vi "FPGA Server v2.vi"() -> ()   [LabVIEW 2013]
doc: "This is the FPGA server for the sbRIO for the open-path cavity ring down."
uses:
  <vilib>/eio/EIONode/EIONode.xnode
  <vilib>/rvi/eio/common/nirviEmuTemplateMethod_errors.vi
  <vilib>/rvi/DataTransferAndStorage/Container/XNode/niFpgaContainer.xnode
  <vilib>/Platform/TimedLoop/XDataNode/XDataNode.xnode
  <vilib>/Platform/TimedLoop/XDataNode/nitl_modes.ctl
  <vilib>/Platform/TimedLoop/XDataNode/XDNodeRunTimeDep.lvlib
  <vilib>/Platform/TimedLoop/XDataNode/wakeup.ctl
  <vilib>/Platform/TimedLoop/XDataNode/timing_clust.ctl
  <vilib>/rvi/Memory/Memory_Emulation/nirvimemoryFastEmulation.vi
  <vilib>/rvi/Memory/Memory_Emulation/nirvimemoryEmulation.vi
  <vilib>/rvi/FIFO/Fifo_Resource/nirvififoEmulationRead.vi
  <vilib>/rvi/FIFO/Fifo_Resource/nirvififoEmulationWrite.vi
  <vilib>/rvi/interface/RandomDataEmulation/nirviRandomDataFpgaReadWriteTemplate.vi
  <vilib>/rvi/FXPMathLib/FxpMul/XNode/nifxpmath_Multiplier.xnode
  <vilib>/rvi/FXPMathLib/sim/FxpSim.dll
panel:
  out "LaserOFF?":bool
  in  "Cylce (ticks)":u32=40000
  in  "Sample (ticks)":u32=8000
  out "DataRead":bool
  out "dataready":bool
  out "NewData":u16
  out "NumElements":u32
  out "Samps":u64
  in  "Stop":bool
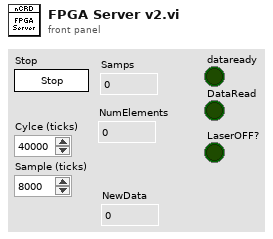
[diagram p1: front panel]
types:
  T1 = typedef "XDNodeRunTimeDep.lvlib/timing_clust.ctl" = cluster{"Expected End [f-1]":u64, "Actual End [f-1]":u64, "Finished Late? [f-1]":bool, "Expected End [i-1]":u64, "Actual End [i-1]":u64, "Finished Late? [i-1]":bool, "Expected Start [i]":u64, "Actual Start [i]":u64, "Expected Start [f]":u64, "Actual Start [f]":u64, "Source Name":string, "Structure Name":string, "Period":i64, "Deadline":i64, "Offset":i64, "Start":i64, "Priority":i32, "Timeout":i32, "Mode":T2, "Wakeup Reason":T3, "Error":errorcluster, "Source Type":string, "Secondary Source Type":string, "Global End Time":u64, "Global Start Time":u64, "Frame Duration":u64, "Iteration Duration":u64, "Assigned CPU":i32, "I/O Scan Engine Mode":u32}
  T2 = typedef "XDNodeRunTimeDep.lvlib/nitl_modes.ctl" = enum32{"No Change", "Process missed periods, maintain original phase", "Discard missed periods, maintain original phase", "Process missed periods, ignore original phase", "Discard missed periods, ignore original phase"}
  T3 = typedef "XDNodeRunTimeDep.lvlib/wakeup.ctl" = enum32{"Normal", "Aborted", "Asynchronous wakeup", "Timing source error", "Timed loop error", "Timeout"}
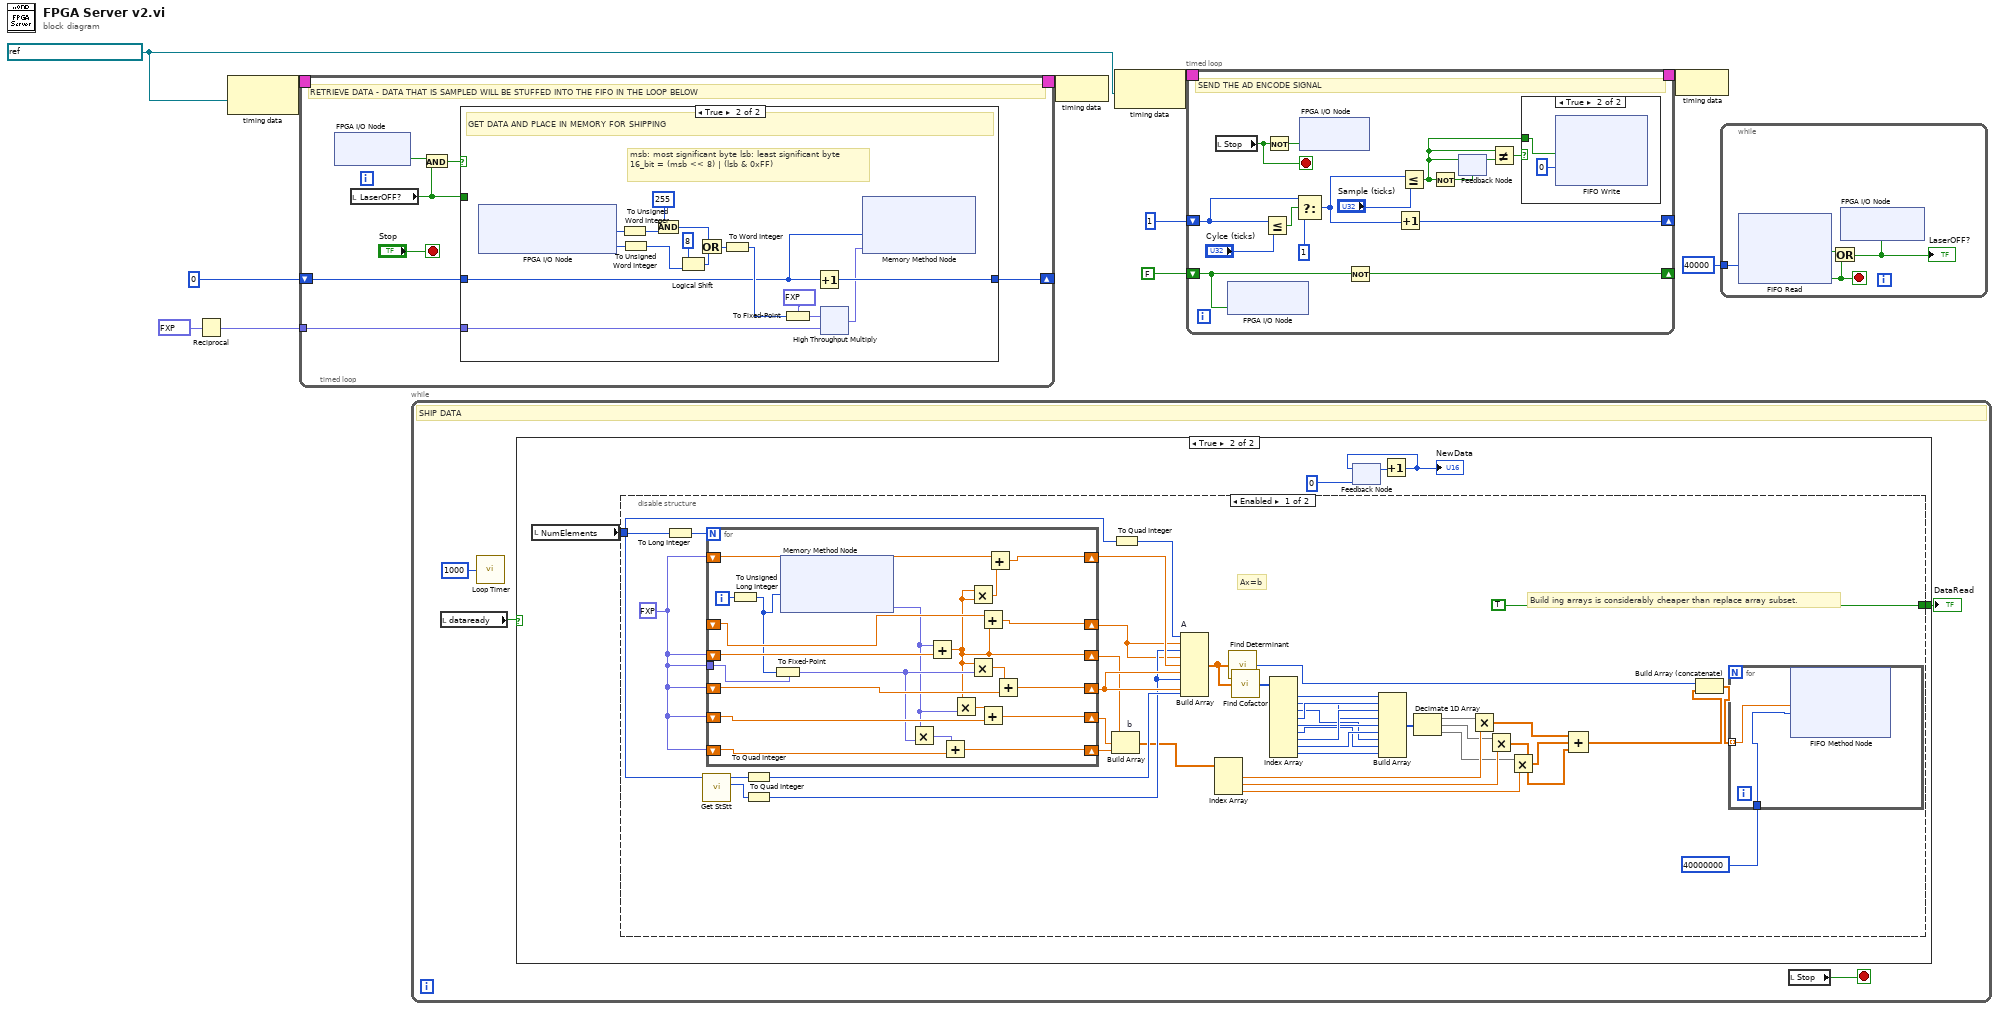
[diagram p0: block diagram]
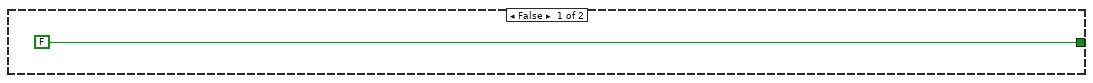
[diagram p2: hidden frame]
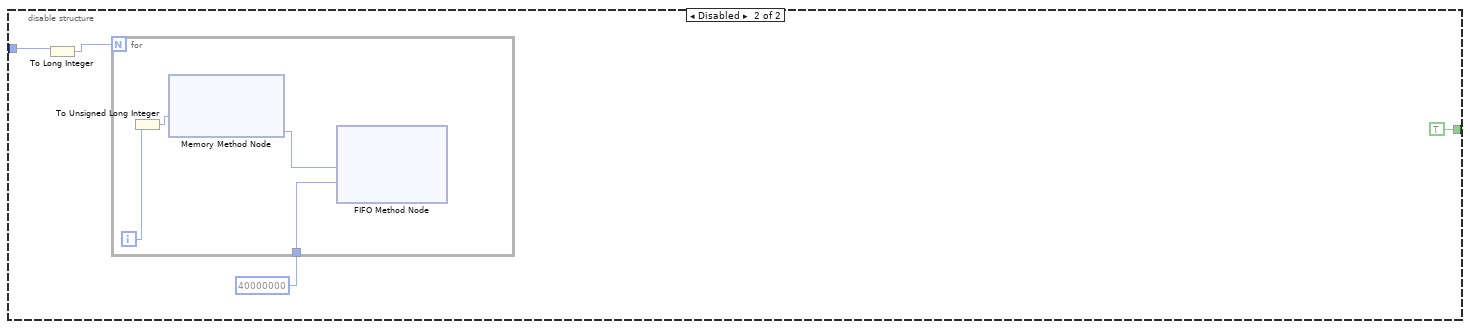
[diagram p3: hidden frame]
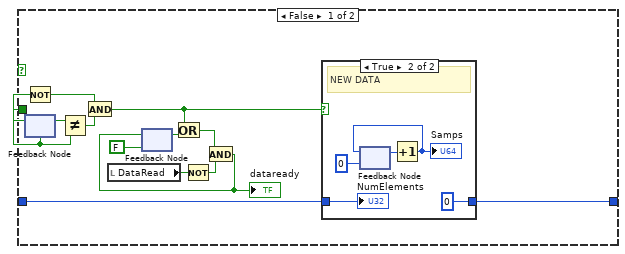
[diagram p4: hidden frame]
diagram:
  w6 = refnum<k21> "40 MHz Onboard Clock" ("Source Name")
  n1 = Reciprocal(x=fxp<+,16,16> 65535.0) -> (1/x=w1:fxp<+/-,32,1>)
  n2 = node-c288(w6) -> (w9:T1)
  n3 = timed-loop {
    timing: w9 -> [_]
    timing-out: [_] -> w8
    shift-right: [w15] -> _
    shift-left: u32 0 -> [w16]
    tunnel: w1 -> [w12]
    stop <- "Stop" stop-if-true
    # "RETRIEVE DATA - DATA THAT IS SAMPLED WILL BE STUFFED INTO THE FIFO IN THE LOOP BELOW"
    n4 = xnode "FPGA I/O Node"() -> ("AD CLK"=w13:bool)  [unwired: 1 in, 1 out]
    n5 = local read "LaserOFF?"() -> (w14:bool)
    n6 = And(x=w13, y=w14) -> (x .and. y?=w17:bool)
    n7 = case shown="True" w17 {
      tunnel: w14 -> [w30 _]
      tunnel: w16 -> [w27 w38]
      tunnel: [w26 w44] -> w15
      tunnel: w12 -> [_ w43]
      frame False {
        n8 = Not(x=w30) -> (.not. x?=w28:bool)
        n9 = feedback-in #1(w30) -> ()
        n10 = feedback #1(w30) -> (w31:bool)
        n11 = Not Equal?(x=w31, y=w30) -> (x != y?=w29:bool)
        n12 = And(x=w28, y=w29) -> (x .and. y?=w22:bool)
        n13 = local read "DataRead"() -> (w23:bool)
        n14 = feedback #2(FALSE) -> (w21:bool)
        n15 = Or(x=w22, y=w21) -> (x .or. y?=w20:bool)
        n16 = Not(x=w23) -> (.not. x?=w24:bool)
        n17 = And(x=w20, y=w24) -> (x .and. y?=w19:bool)
        "dataready" <- w19
        n18 = feedback-in #2(w19) -> ()
        n19 = case shown="True" w22 {
          tunnel: w27 -> [w32 w33]
          tunnel: [w32 u32 0] -> w26
          frame False {
          }
          frame True {
            # "NEW DATA"
            n20 = feedback #3(u64 0) -> (w36:u64)
            n21 = Increment(x=w36) -> (x+1=w35:u64)
            "Samps" <- w35
            n22 = feedback-in #3(w35) -> ()
            "NumElements" <- w33
          }
        }
      }
      frame True {
        # "msb: most significant byte lsb: least significant byte 16_bit = (msb << 8) | (lsb & 0xFF)"
        # "GET DATA AND PLACE IN MEMORY FOR SHIPPING"
        n23 = xnode "FPGA I/O Node"() -> ("RMC/LVTTL/DIO7:0"=w52:u8, "RMC/LVTTL/DIO15:8"=w53:u8)  [unwired: 2 in, 2 out]
        n24 = To Unsigned Word Integer(number=w52) -> (unsigned 16bit integer=w46:u16)
        n25 = To Unsigned Word Integer(number=w53) -> (unsigned 16bit integer=w48:u16)
        n26 = And(x=u16 255 ("y"), y=w46) -> (x .and. y?=w50:u16)
        n27 = Logical Shift(y=i16 8, x=w48) -> (x << y=w49:u16)
        n28 = Or(x=w50, y=w49) -> (x .or. y?=w45:u16)
        n29 = To Word Integer(number=w45) -> (16bit integer=w41:i16)
        n30 = To Fixed-Point(fixed-point type=fxp<+,16,16> 32767.0, number=w41) -> (fixed-point=w40:fxp<+,16,16>)
        n31 = Increment(x=w38) -> (x+1=w44:u32)
        n32 = xnode "High Throughput Multiply"("x"=w40, "y"=w43) -> ("x*y"=w39:fxp<+,16,1>)
        n33 = xnode ("Memory Method Node")("Address"=w38, "Data"=w39) -> ()  [unwired: 1 in, 1 out]
      }
    }
  }
  n34 = while {
    stop <- w59 stop-if-true
    # "SHIP DATA"
    n35 = local read "dataready"() -> (w58:bool)
    n36 = call "Loop Timer"("Count(Ticks)"=u32 1000) -> ()  [unwired: 1 out]
    n37 = case shown="True" w58 {
      tunnel: [FALSE w65] -> w57
      frame False {
      }
      frame True {
        n38 = local read "NumElements"() -> (w64:u32)
        n39 = disable-structure shown="Enabled" {
          disable-tunnel: [TRUE TRUE] -> w65
          disable-tunnel: w64 -> [w94 w131]
          frame Enabled {
            w66 = fxp<+,16,1> 0.0 ("x*y")
            # "Ax=b"
            # "Build ing arrays is considerably cheaper than replace array subset."
            n40 = To Long Integer(number=w94) -> (32bit integer=w105:i32)
            n41 = call "Get StStt.vi"("N"=w94) -> ("St"=w95:u32, "Stt"=w96:u32)  [unwired: 9 in]
            n42 = for {
              N: w105 -> [_]
              shift-right: [w116] -> w99
              shift-left: w66 -> [w126]
              shift-right: [w115] -> w104
              shift-left: w66 -> [w125]
              shift-right: [w123] -> w103
              shift-left: w66 -> [w124]
              shift-right: [w122] -> w98
              shift-left: w66 -> [w121]
              shift-right: [w119] -> w97
              shift-left: w66 -> [w118]
              shift-right: [w114] -> w92
              shift-left: _ -> [w117]
              tunnel: w66 -> [w107]
              i -> [w127]
              n43 = To Unsigned Long Integer(number=w127) -> (unsigned 32bit integer=w109:u32)
              n44 = To Fixed-Point(fixed-point type=w107, number=w109) -> (fixed-point=w120:fxp<+,16,1>)
              n45 = xnode ("Memory Method Node")("Address"=w109) -> ("Data"=w108:fxp<+,16,1>)  [unwired: 1 in, 1 out]
              n46 = Multiply(x=w108, y=w120) -> (x*y=w110:fxp<+,32,2>)
              n47 = Add(x=w108, y=w126) -> (x+y=w116:dbl)
              n48 = Add(x=w110, y=w118) -> (x+y=w119:dbl)
              n49 = Multiply(x=w116, y=w108) -> (x*y=w111:dbl)
              n50 = Multiply(x=w116, y=w116) -> (x*y=w113:dbl)
              n51 = Multiply(x=w116, y=w120) -> (x*y=w112:dbl)
              n52 = Add(x=w117, y=w116) -> (x+y=w114:dbl)
              n53 = Add(x=w111, y=w121) -> (x+y=w122:dbl)
              n54 = Add(x=w125, y=w113) -> (x+y=w115:dbl)
              n55 = Add(x=w112, y=w124) -> (x+y=w123:dbl)
            }
            n56 = To Quad Integer(1:w96) -> (0:w102:i64)
            n57 = To Quad Integer(1:w95) -> (0:w101:i64)
            n58 = Build Array "b"(w99, w98, w97) -> (w80:dbl[])
            n59 = To Quad Integer(1:w94) -> (0:w93:i64)
            n60 = Build Array "A"(w93, w92, w101, w92, w104, w103, w101, w103, w102) -> (w100:dbl[])
            n61 = Index Array(array=w80) -> (element #1=w78:dbl, element #2=w76:dbl, element #3=w74:dbl)  [unwired: 3 in]
            n62 = call "Find Determinant.vi"("A"=w100) -> ("det(A)"=w68:i64)  [unwired: 4 in]
            n63 = call "Find Cofactor.vi"("A"=w100) -> ("cofA"=w91:i64[])  [unwired: 4 in]
            n64 = Index Array(array=w91) -> (element #1=w90:i64, element #2=w87:i64, element #3=w84:i64, element #4=w89:i64, element #5=w86:i64, element #6=w83:i64, element #7=w88:i64, element #8=w85:i64, element #9=w82:i64)  [unwired: 9 in]
            n65 = Build Array(w90, w89, w88, w87, w86, w85, w84, w83, w82) -> (w81:i64[])
            n66 = Decimate 1D Array(w81) -> (w79:i64[], w77:i64[], w75:i64[])
            n67 = Multiply(x=w79, y=w78) -> (x*y=w73:dbl[])
            n68 = Multiply(x=w77, y=w76) -> (x*y=w71:dbl[])
            n69 = Multiply(x=w75, y=w74) -> (x*y=w72:dbl[])
            n70 = Compound Arithmetic op=ADD(w73, w72, w71) -> (w69:dbl[])
            n71 = Build Array (concatenate)(w68, w69) -> (w67:dbl[])
            n72 = for {
              tunnel: w67 -> [w128] mode=indexing
              tunnel: 40000000 ("Timeout") -> [w129]
              n73 = xnode ("FIFO Method Node")("Element"=w128, "Timeout"=w129) -> ()  [unwired: 1 in, 2 out]
            }
          }
          frame Disabled {
            n74 = To Long Integer(number=w131) -> (32bit integer=w130:i32)
            n75 = for {
              N: w130 -> [_]
              tunnel: 40000000 ("Timeout") -> [w136]
              i -> [w135]
              n76 = To Unsigned Long Integer(number=w135) -> (unsigned 32bit integer=w134:u32)
              n77 = xnode ("Memory Method Node")("Address"=w134) -> ("Data"=w137:i16)  [unwired: 1 in, 1 out]
              n78 = xnode ("FIFO Method Node")("Element"=w137, "Timeout"=w136) -> ()  [unwired: 1 in, 2 out]
            }
          }
        }
        n79 = feedback #4(u16 0) -> (w62:u16)
        n80 = Increment(x=w62) -> (x+1=w63:u16)
        "NewData" <- w63
        n81 = feedback-in #4(w63) -> ()
      }
    }
    "DataRead" <- w57
    n82 = local read "Stop"() -> (w59:bool)
  }
  n83 = node-c288(w8) -> ()
  n84 = node-c288(w6) -> (w11:T1)
  n85 = timed-loop {
    shift-right: [w152] -> _
    shift-left: FALSE -> [w151]
    timing: w11 -> [_]
    timing-out: [_] -> w10
    shift-right: [w142] -> _
    shift-left: u32 1 -> [w143]
    stop <- w149 stop-if-true
    # "SEND THE AD ENCODE SIGNAL"
    n86 = local read "Stop"() -> (w149:bool)
    n87 = xnode "FPGA I/O Node"("ENCODE"=w151) -> ()  [unwired: 1 in, 1 out]
    n88 = Less Or Equal?(x=w143, y="Cylce (ticks)") -> (x <= y?=w147:bool)
    n89 = Not(x=w149) -> (.not. x?=w150:bool)
    n90 = Select(t=w143, s=w147, f=u32 1) -> (s? t:f=w144:u32)
    n91 = xnode "FPGA I/O Node"("AD EN"=w150) -> ()  [unwired: 1 in, 1 out]
    n92 = Not(x=w151) -> (.not. x?=w152:bool)
    n93 = Increment(x=w144) -> (x+1=w142:u32)
    n94 = Less Or Equal?(x=w144, y="Sample (ticks)") -> (x <= y?=w138:bool)
    n95 = Not(x=w138) -> (.not. x?=w141:bool)
    n96 = feedback-in #5(w138) -> ()
    n97 = feedback #5(w141) -> (w140:bool)
    n98 = Not Equal?(x=w138, y=w140) -> (x != y?=w139:bool)
    n99 = case shown="True" w139 {
      tunnel: w138 -> [_ w154]
      frame False {
      }
      frame True {
        n100 = xnode ("FIFO Write")("Element"=w154, "Timeout"=0) -> ()  [unwired: 1 in, 2 out]
      }
    }
  }
  n101 = node-c288(w10) -> ()
  n102 = while {
    tunnel: 40000 ("Timeout") -> [w157]
    stop <- w158 stop-if-true
    n103 = xnode ("FIFO Read")("Timeout"=w157) -> ("Element"=w160:bool, "Timed Out?"=w158:bool)  [unwired: 1 in, 1 out]
    n104 = Or(x=w160, y=w158) -> (x .or. y?=w159:bool)
    "LaserOFF?" <- w159
    n105 = xnode "FPGA I/O Node"("Laser Out"=w159) -> ()  [unwired: 1 in, 1 out]
  }
